vi "Stop Log.vi"(8 "error in (no error)":errorcluster, 11 "Data Logger Module in":refnum<class "Data Logger Module.lvclass">) -> (0 "error out":errorcluster, 3 "Data Logger Module out":refnum<class "Data Logger Module.lvclass">)   [LabVIEW 2020, in "VolatusData.lvlib" / "Data Logger Module.lvclass"]
uses:
  Data Logger Module.lvclass
  Data Logger Module.lvclass/Data Logger Module.ctl
  Logger Stopped.ctl
  Volatus/MessageQ/MessageQ.lvclass/MessageQ.ctl
  Volatus/MessageQ/MessageQ.lvclass
  VolatusData.lvlib
  Logger State.ctl
  C:/dev/lv20CE/relink/lv-volatus/Volatus/Module/Module.lvclass
  C:/dev/lv20CE/relink/lv-volatus/VolatusData/Data Logger Module/Data Logger Module.lvclass
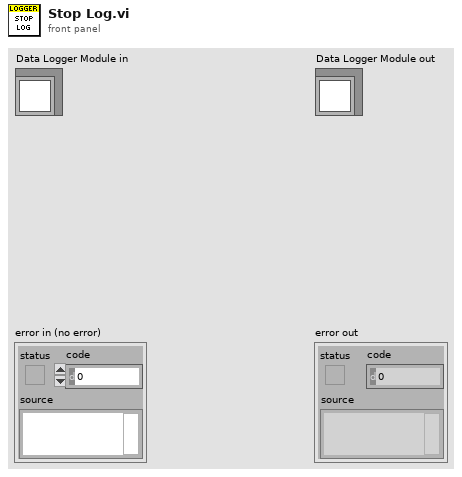
[diagram p1: front panel]
types:
  T1 = typedef "VolatusData.lvlib/Logger State.ctl" = enum16{"Unknown", "Idle", "Preparing", "Ready", "Logging", "Stopping"}
  T2 = typedef "VolatusData.lvlib/Logger Stopped.ctl" = cluster{"ID":string}
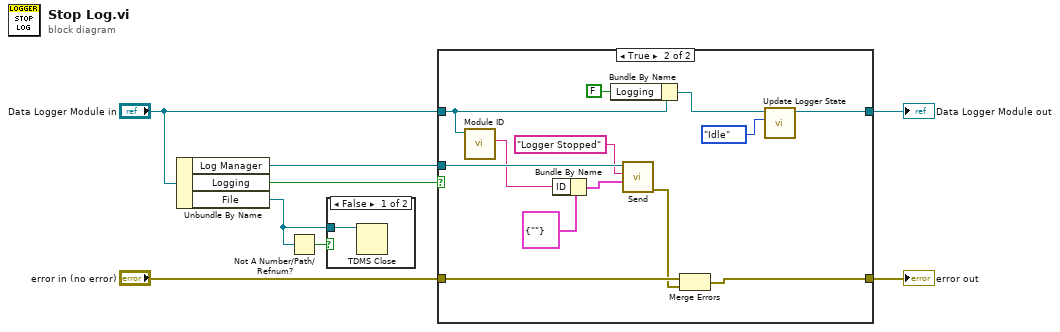
[diagram p0: block diagram]
diagram:
  n1 = Unbundle By Name("Data Logger Module in") -> ("Log Manager"=w3:refnum<class "MessageQ.lvclass">, "Logging"=w6:bool, "File"=w7:refnum<k34>)
  n2 = Not A Number/Path/Refnum?(number/path/refnum=w7) -> (NaN/Path/Refnum?=w8:bool)
  n3 = case shown="False" w8 {
    tunnel: w7 -> [w9 _]
    frame False {
      n4 = TDMS Close(11:w9) -> ()  [unwired: 1 in, 2 out]
    }
    frame True {
    }
  }
  n5 = case shown="True" w6 {
    tunnel: "error in (no error)" -> [w11 w19]
    tunnel: "Data Logger Module in" -> [w10 w16]
    tunnel: w3 -> [_ w24]
    tunnel: [w11 w17] -> w2
    tunnel: [w10 w13] -> w1
    frame False {
    }
    frame True {
      n6 = call-dynamic "Module ID.vi"("Data Logger Module in"=w16) -> ("Module ID"=w20:string)  [unwired: 10 in]
      n7 = Bundle By Name(cluster=T2 {"ID"=""} ("Logger Stopped"), "ID"=w20) -> (w22:T2)
      n8 = Bundle By Name(cluster=w16, "Logging"=FALSE) -> (w14:refnum<class "Data Logger Module.lvclass">)
      n9 = call "Send.vi"("Data"=w22, "ID"="Logger Stopped", "MessageQ in"=w24) -> ("error out"=w18:errorcluster)  [unwired: 7 in, 1 out]
      n10 = Merge Errors(w19, w18) -> (w17:errorcluster)
      n11 = call "Update Logger State.vi"("Logger State"=Logger_State."Idle", "Module in"=w14) -> ("Module"=w13:refnum<class "Data Logger Module.lvclass">)  [unwired: 8 in, 1 out]
    }
  }
  "error out" <- w2
  "Data Logger Module out" <- w1
